vi "Schedsteptodisplay.vi"(10 "step num":u32, 11 "step array":string[](array[string])) -> (2 "STEP VARS":T1)   [LabVIEW 2023]
uses:
  stepvariables.ctl
panel:
  # "STEP"
  # "NAME"
  # "NOTES"
  # "PARAMS"
  # "KV SP"
  # "KV RDG"
  # "MA/IF SP"
  # "MA/IF RDG"
  # "EXP sec SP"
  # "EXP sec RDG"
  # "COOL sec SP"
  # "COOL sec RDG"
  # "scans.Mode"
  # "data item"
  # "min"
  # "max"
  # "init BIAS SP"
  # "init BIAS RDG"
  # "init DIFF SP"
  # "max Gx"
  # "init EfDr SP"
  # "init EfDr RDG"
  # "max Tries"
  # "TEST"
  # "LIM1"
  # "LIM2"
  # "LIM4"
  # "LIM3"
  # "CHAIN SCHEDS"
  # "RPTS"
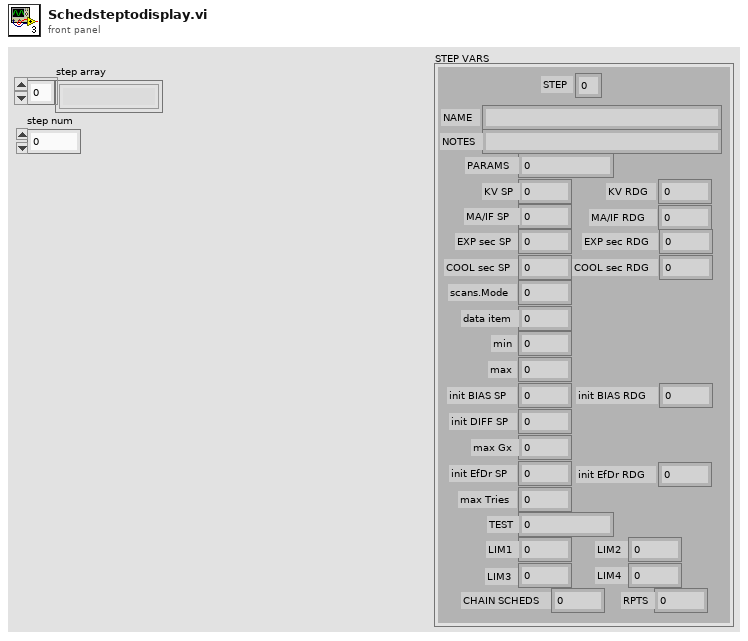
[diagram p1: front panel]
types:
  T1 = typedef "stepvariables.ctl" = cluster{"NAME":string, "NOTES":string, "PARAMS":u32, "KV  SP":dbl, "KV  RDG":dbl, "MA/IF  SP":dbl, "MA/IF  RDG":dbl, "init BIAS SP":dbl, "init BIAS RDG":dbl, "max Gx":dbl, "TEST":u32, "min":dbl, "max":dbl, "LIM1":dbl, "LIM2":dbl, "LIM3":dbl, "LIM4":dbl, "data item":dbl, "chain scheds":dbl, "REPEATS":dbl, "STEP NUM":u32, "EXP s SP":dbl, "EXP s RDG":dbl, "COOL s SP":dbl, "COOL s RDG":dbl, "scans mode":dbl, "init EfDr":dbl, "init EfDr RDG":dbl, "max Tries":dbl, "init DIFF SP":dbl}
  T2 = cluster{"step array[0]":string, "step array[1]":string, "step array[2]":string, "step array[3]":string, "step array[4]":string, "step array[5]":string, "step array[6]":string, "step array[7]":string, "step array[8]":string, "step array[9]":string, "step array[10]":string, "step array[11]":string, "step array[12]":string, "step array[13]":string, "step array[14]":string, "step array[15]":string, "step array[16]":string, "step array[17]":string, "step array[18]":string, "step array[19]":string, "step array[20]":string}
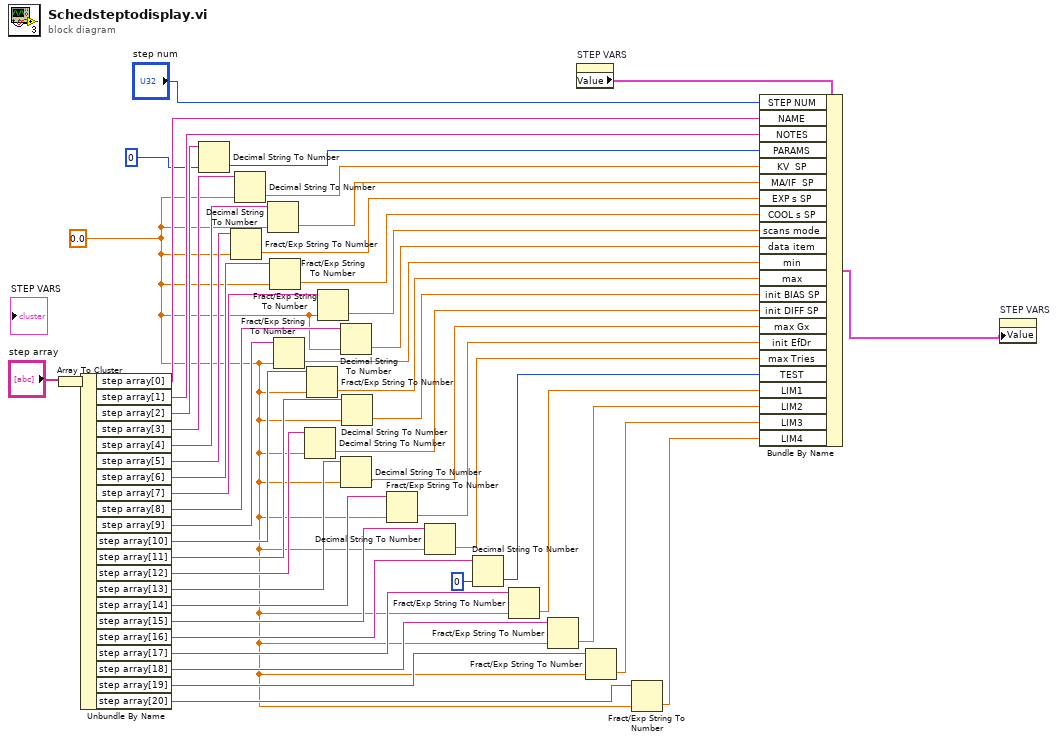
[diagram p0: block diagram]
diagram:
  w5 = 0.0 ("default (0 I32)")
  n1 = Array To Cluster(array="step array") -> (cluster=w47:T2)
  n2 = Unbundle By Name(w47) -> ("step array[0]"=w46:string, "step array[1]"=w45:string, "step array[2]"=w44:string, "step array[3]"=w42:string, "step array[4]"=w41:string, "step array[5]"=w40:string, "step array[6]"=w39:string, "step array[7]"=w38:string, "step array[8]"=w37:string, "step array[9]"=w36:string, "step array[10]"=w35:string, "step array[11]"=w34:string, "step array[12]"=w22:string, "step array[13]"=w20:string, "step array[14]"=w31:string, "step array[15]"=w14:string, "step array[16]"=w13:string, "step array[17]"=w12:string, "step array[18]"=w11:string, "step array[19]"=w10:string, "step array[20]"=w7:string)
  n3 = Decimal String To Number(string=w44, default (0L)=u32 0 ("default (0 I32)")) -> (number=w43:u32)  [unwired: 1 in, 1 out]
  n4 = Fract/Exp String To Number(string=w40, default (0 dbl)=w5) -> (number=w29:dbl)  [unwired: 2 in, 1 out]
  n5 = Decimal String To Number(string=w42, default (0L)=w5) -> (number=w33:dbl)  [unwired: 1 in, 1 out]
  n6 = Decimal String To Number(string=w41, default (0L)=w5) -> (number=w32:dbl)  [unwired: 1 in, 1 out]
  n7 = Fract/Exp String To Number(string=w39, default (0 dbl)=w5) -> (number=w28:dbl)  [unwired: 2 in, 1 out]
  n8 = Fract/Exp String To Number(string=w36, default (0 dbl)=w5) -> (number=w25:dbl)  [unwired: 2 in, 1 out]
  n9 = Decimal String To Number(string=w22, default (0L)=w5) -> (number=w21:dbl)  [unwired: 1 in, 1 out]
  n10 = Fract/Exp String To Number(string=w35, default (0 dbl)=w5) -> (number=w24:dbl)  [unwired: 2 in, 1 out]
  n11 = Fract/Exp String To Number(string=w38, default (0 dbl)=w5) -> (number=w27:dbl)  [unwired: 2 in, 1 out]
  n12 = Decimal String To Number(string=w37, default (0L)=w5) -> (number=w26:dbl)  [unwired: 1 in, 1 out]
  n13 = Decimal String To Number(string=w20, default (0L)=w5) -> (number=w19:dbl)  [unwired: 1 in, 1 out]
  n14 = Decimal String To Number(string=w34, default (0L)=w5) -> (number=w23:dbl)  [unwired: 1 in, 1 out]
  n15 = Fract/Exp String To Number(string=w31, default (0 dbl)=w5) -> (number=w18:dbl)  [unwired: 2 in, 1 out]
  n16 = Decimal String To Number(string=w14, default (0L)=w5) -> (number=w17:dbl)  [unwired: 1 in, 1 out]
  n17 = Decimal String To Number(string=w13, default (0L)=u32 0 ("default (0 I32)")) -> (number=w16:u32)  [unwired: 1 in, 1 out]
  n18 = Fract/Exp String To Number(string=w12, default (0 dbl)=w5) -> (number=w15:dbl)  [unwired: 2 in, 1 out]
  n19 = Fract/Exp String To Number(string=w11, default (0 dbl)=w5) -> (number=w9:dbl)  [unwired: 2 in, 1 out]
  n20 = property on="STEP VARS" class="Clust (strict)"() -> ("Value"=w2:T1)  [unwired: 2 in, 2 out]
  n21 = Fract/Exp String To Number(string=w10, default (0 dbl)=w5) -> (number=w8:dbl)  [unwired: 2 in, 1 out]
  n22 = Fract/Exp String To Number(string=w7, default (0 dbl)=w5) -> (number=w6:dbl)  [unwired: 2 in, 1 out]
  n23 = Bundle By Name(cluster=w2, "STEP NUM"="step num", "NAME"=w46, "NOTES"=w45, "PARAMS"=w43, "KV  SP"=w33, "MA/IF  SP"=w32, "EXP s SP"=w29, "COOL s SP"=w28, "scans mode"=w27, "data item"=w26, "min"=w25, "max"=w24, "init BIAS SP"=w23, "init DIFF SP"=w21, "max Gx"=w19, "init EfDr"=w18, "max Tries"=w17, "TEST"=w16, "LIM1"=w15, "LIM2"=w9, "LIM3"=w8, "LIM4"=w6) -> (w1:T1)
  n24 = property on="STEP VARS" class="Clust (strict)"("Value"=w1) -> ()  [unwired: 2 in, 2 out]
